vi "PathTest.vi"() -> ()   [LabVIEW 2023]
panel:
  out "Path 3":path
  out "Path 2":path
  out "Path":path
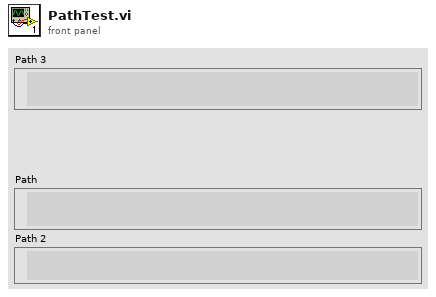
[diagram p1: front panel]
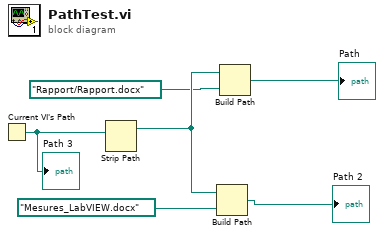
[diagram p0: block diagram]
diagram:
  n1 = Current VI's Path() -> (path=w1:path)
  "Path 3" <- w1
  n2 = Strip Path(path=w1) -> (stripped path=w6:path)  [unwired: 1 out]
  n3 = Build Path(base path=w6, name or relative path=path "Mesures_LabVIEW.docx") -> (appended path=→"Path 2":path)
  n4 = Build Path(base path=w6, name or relative path=path "Rapport/Rapport.docx") -> (appended path=→"Path":path)
